vi "Parse One DBL Arg.vi"(9 "State String":string) -> (1 "Numeric Arg":dbl)   [LabVIEW 2013]
doc: "This sub-VI parses a single numeric argument from an input string with the format \"state:arg\"."
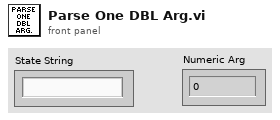
[diagram p1: front panel]
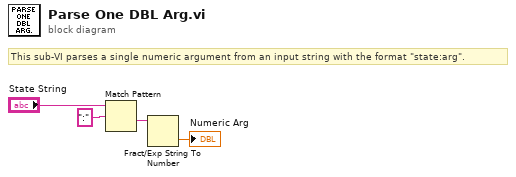
[diagram p0: block diagram]
diagram:
  # "This sub-VI parses a single numeric argument from an input string with the format \"state:arg\"."
  n1 = Match Pattern(string="State String", regular expression=":") -> (after substring=w2:string)  [unwired: 1 in, 3 out]
  n2 = Fract/Exp String To Number(string=w2) -> (number=→"Numeric Arg":dbl)  [unwired: 3 in, 1 out]
